vi "二维数组转一维数组.vi"(1 "表格控件 2":string[][](table) caption="电压采样精度检测") -> (0 "数组":string[](array[string]))   [LabVIEW 2020]
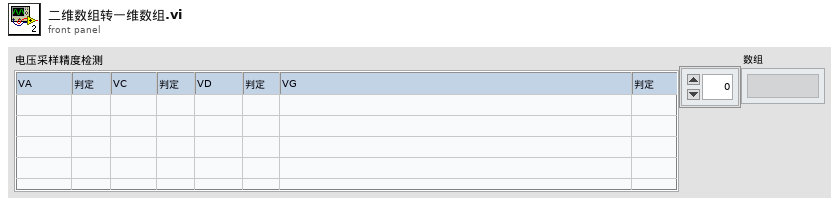
[diagram p1: front panel]
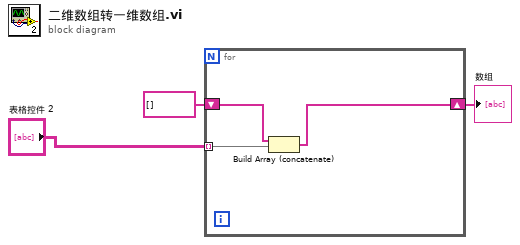
[diagram p0: block diagram]
diagram:
  n1 = for {
    tunnel: "表格控件 2" -> [w6] mode=indexing
    shift-right: [w5] -> w1
    shift-left: string[] [] -> [w4]
    n2 = Build Array (concatenate)(w4, w6) -> (w5:string[])
  }
  "数组" <- w1
